vi "Measurement Logic.vi"() -> ()   [LabVIEW 2021, in "Efficiency And Load Regulation_PMIC.lvlib"]
uses:
  Efficiency And Load Regulation_PMIC.lvlib
  Measurement Configuration.ctl
  Measurement Results.ctl
  <vilib>/Plug-In SDKs/Measurements/Measure Call Context/Measure Call Context.lvclass
  <instrlib>/niDCPower/nidcpower.llb/niDCPower Sense.ctl
  <instrlib>/niDCPower/nidcpower.llb/niDCPower Source Mode.ctl
  <instrlib>/niDCPower/nidcpower.llb/niDCPower Wait For Event - Event.ctl
  <instrlib>/niDCPower/nidcpower.llb/niDCPower Output Function.ctl
  <instrlib>/niDCPower/nidcpower.llb/niDCPower Sequence Attribute Type.ctl
  <instrlib>/niDCPower/nidcpower.llb/niDCPower Get Channel Name From String.vi
  <instrlib>/niDCPower/nidcpower.llb/niDCPower Create Advanced Sequence Step With Channels.vi
  <instrlib>/niDCPower/nidcpower.llb/niDCPower Configure Digital Edge Source Trigger With Channels.vi
  <instrlib>/niDCPower/nidcpower.llb/niDCPower Configure Digital Edge Measure Trigger With Channels.vi
panel:
  out "measure call context out":refnum<class "Measure Call Context.lvclass">
  in  "measure call context in":refnum<class "Measure Call Context.lvclass">
  out "measurement results":T1
  in  "measurement configuration":T2={"Mode of operation"=enum."Perform measurement", "DUT setup time"=1.0, "Source delay"=0.005, "Aperture time"=0.005, "Nominal output voltage"=3.3, "Source resource name"="", "Source current limit"=25.0, "Source maximum power"=300.0, "Source start voltage"=5.0, "Source stop voltage"=20.0, "Source voltage sweep points"=10, "Load resource name"="", "Load voltage limit range"=6.0, "Load sweep type"="Logarithmic", "Load start current"=0.1, "Load stop current"=24.0, "Load current sweep points/points per decade"=10}
  out "error out":errorcluster
  in  "error in":errorcluster
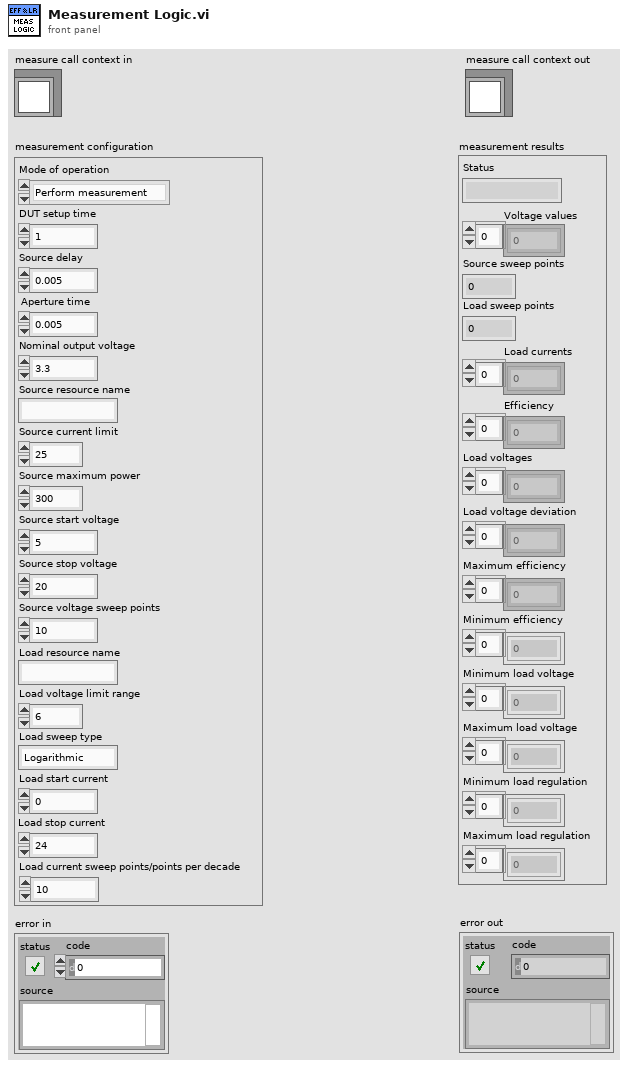
[diagram p1: front panel]
types:
  T1 = typedef "Efficiency And Load Regulation_PMIC.lvlib/Measurement Results.ctl" = cluster{"Status":string, "Voltage values":dbl[], "Source sweep points":i32, "Load sweep points":i32, "Load currents":dbl[], "Efficiency":dbl[], "Load voltages":dbl[], "Load voltage deviation":dbl[], "Maximum efficiency":dbl[], "Minimum efficiency":dbl[], "Minimum load voltage":dbl[], "Maximum load voltage":dbl[], "Minimum load regulation":dbl[], "Maximum load regulation":dbl[]}
  T2 = typedef "Efficiency And Load Regulation_PMIC.lvlib/Measurement Configuration.ctl" = cluster{"Mode of operation":enum32{"Power on the DUT", "Perform measurement", "Power off the DUT"}, "DUT setup time":dbl, "Source delay":dbl, "Aperture time":dbl, "Nominal output voltage":dbl, "Source resource name":string, "Source current limit":dbl, "Source maximum power":dbl, "Source start voltage":dbl, "Source stop voltage":dbl, "Source voltage sweep points":i32, "Load resource name":string, "Load voltage limit range":dbl, "Load sweep type":string, "Load start current":dbl, "Load stop current":dbl, "Load current sweep points/points per decade":i32}
  T3 = cluster{"Voltage values":dbl[], "Source out":refnum<k15>, "Source channel name":string, "Load out":refnum<k15>, "Load channel name":string, "Current values":dbl[], "Load sweep points":i32, "Source terminal name":string, "Measure terminal name":string, "Measurement Results":T1, "Source sequence name":string}
  T4 = enum32{"Power on the DUT", "Perform measurement", "Power off the DUT"}
  T5 = typedef "niDCPower Wait For Event - Event.ctl" = i32
  T6 = typedef "niDCPower Source Mode.ctl" = i32
  T7 = typedef "niDCPower Sense.ctl" = i32
  T8 = typedef "niDCPower Sequence Attribute Type.ctl" = i32
  T9 = typedef "niDCPower Output Function.ctl" = i32
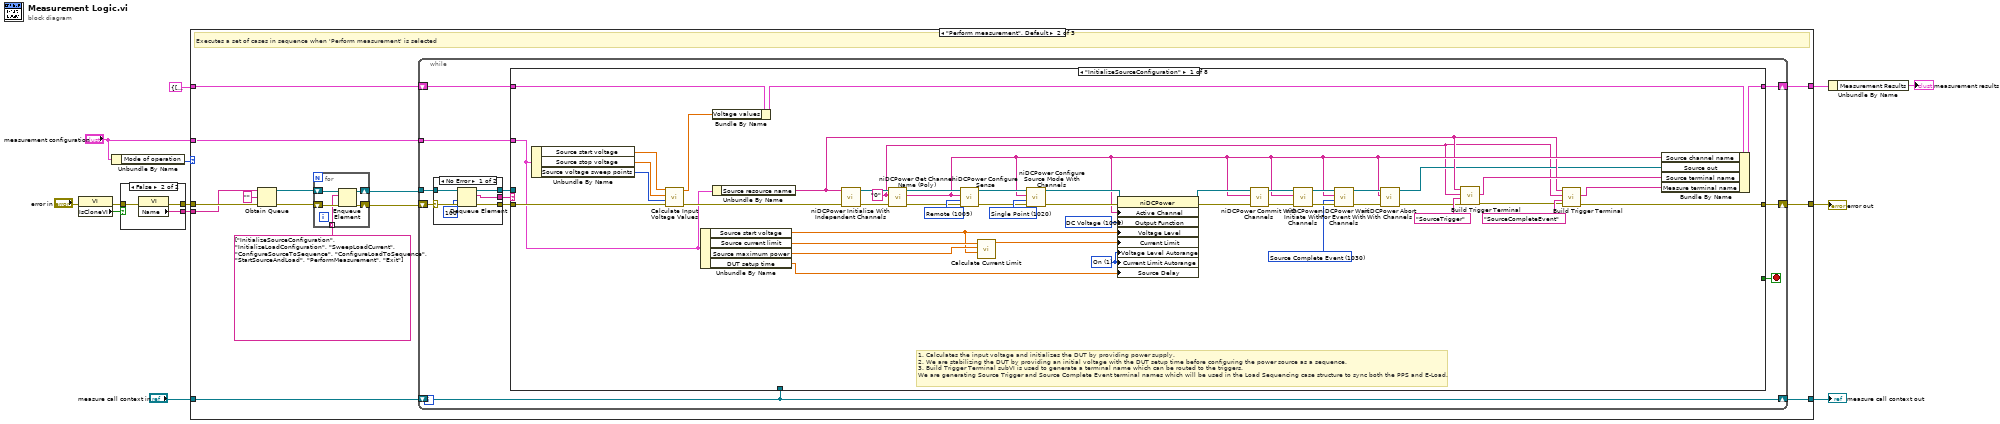
[diagram p0: block diagram]
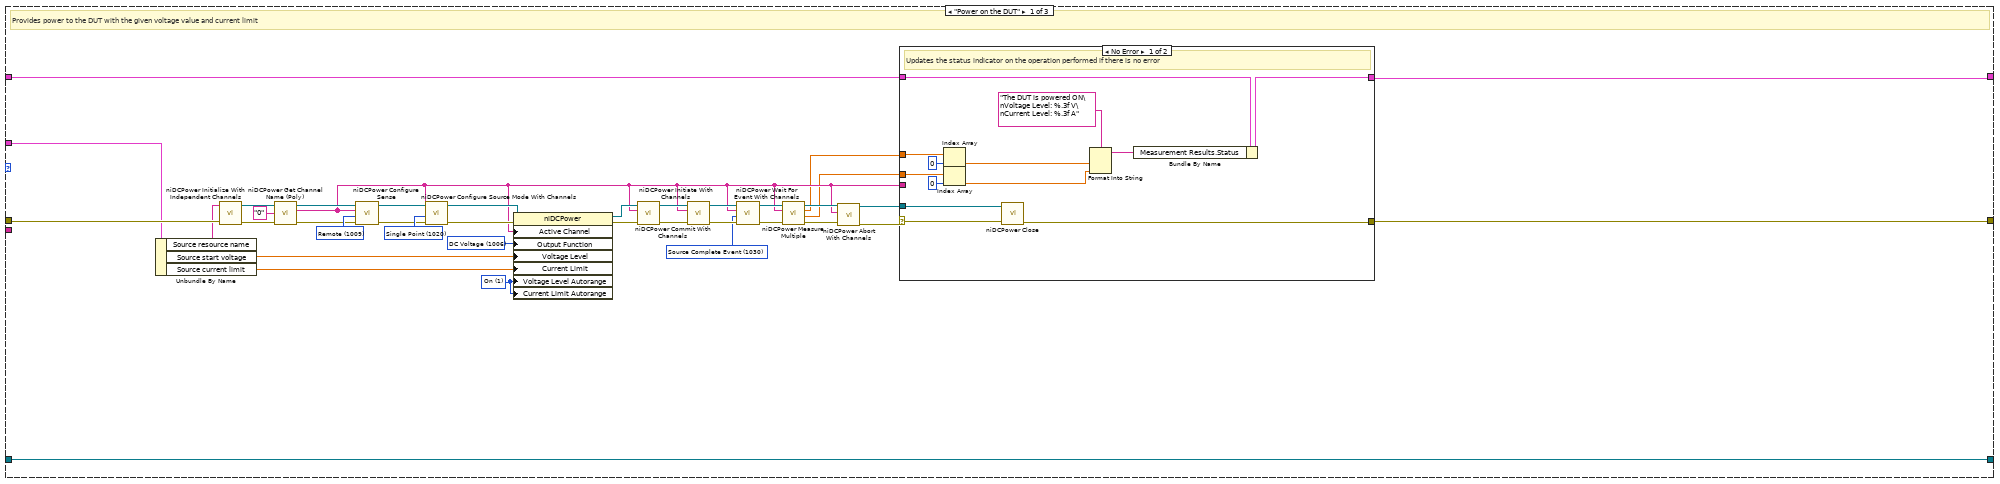
[diagram p2: hidden frame]
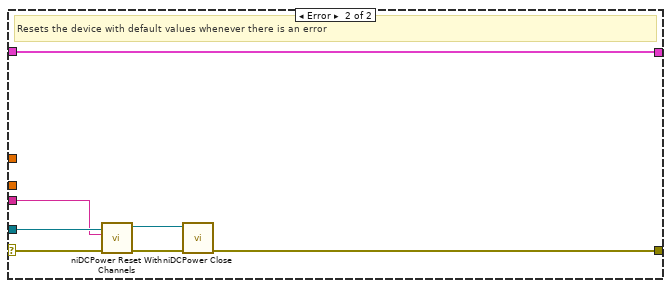
[diagram p3: hidden frame]
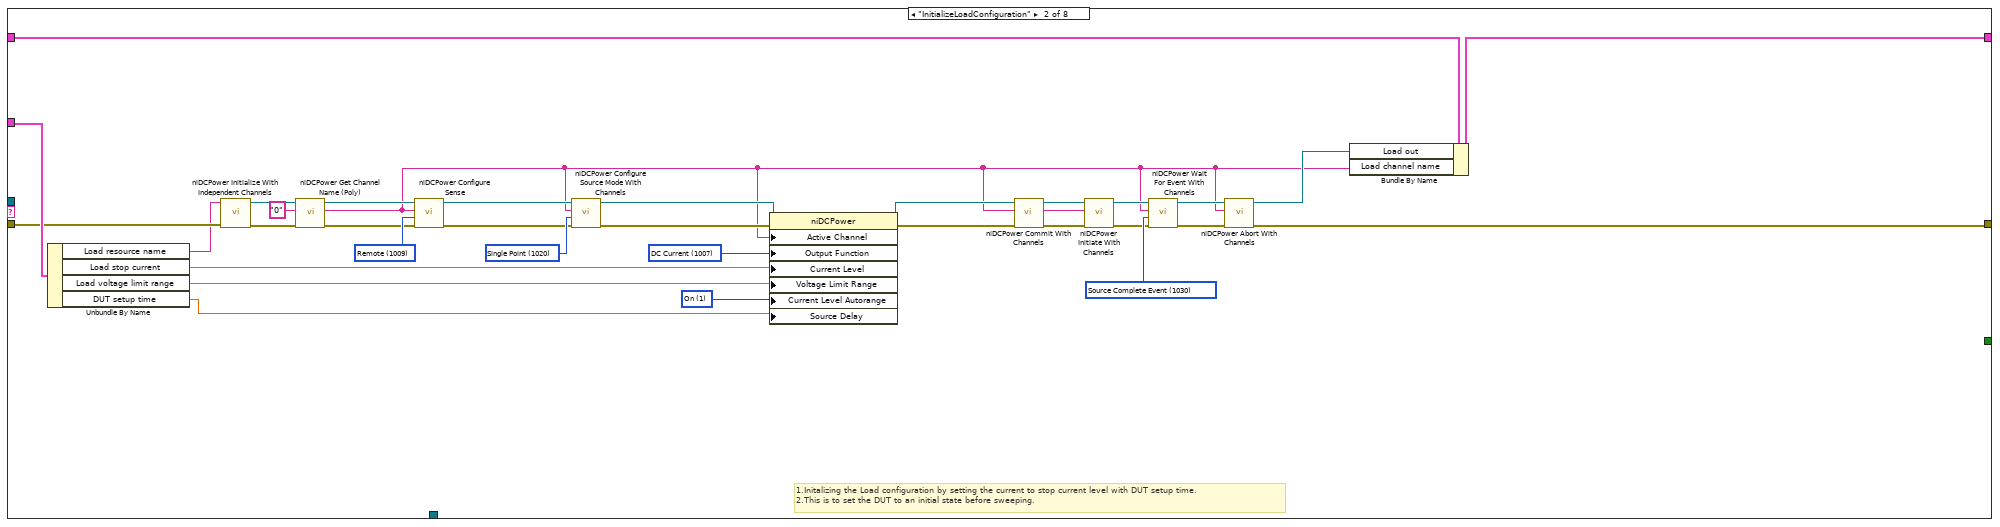
[diagram p4: hidden frame]
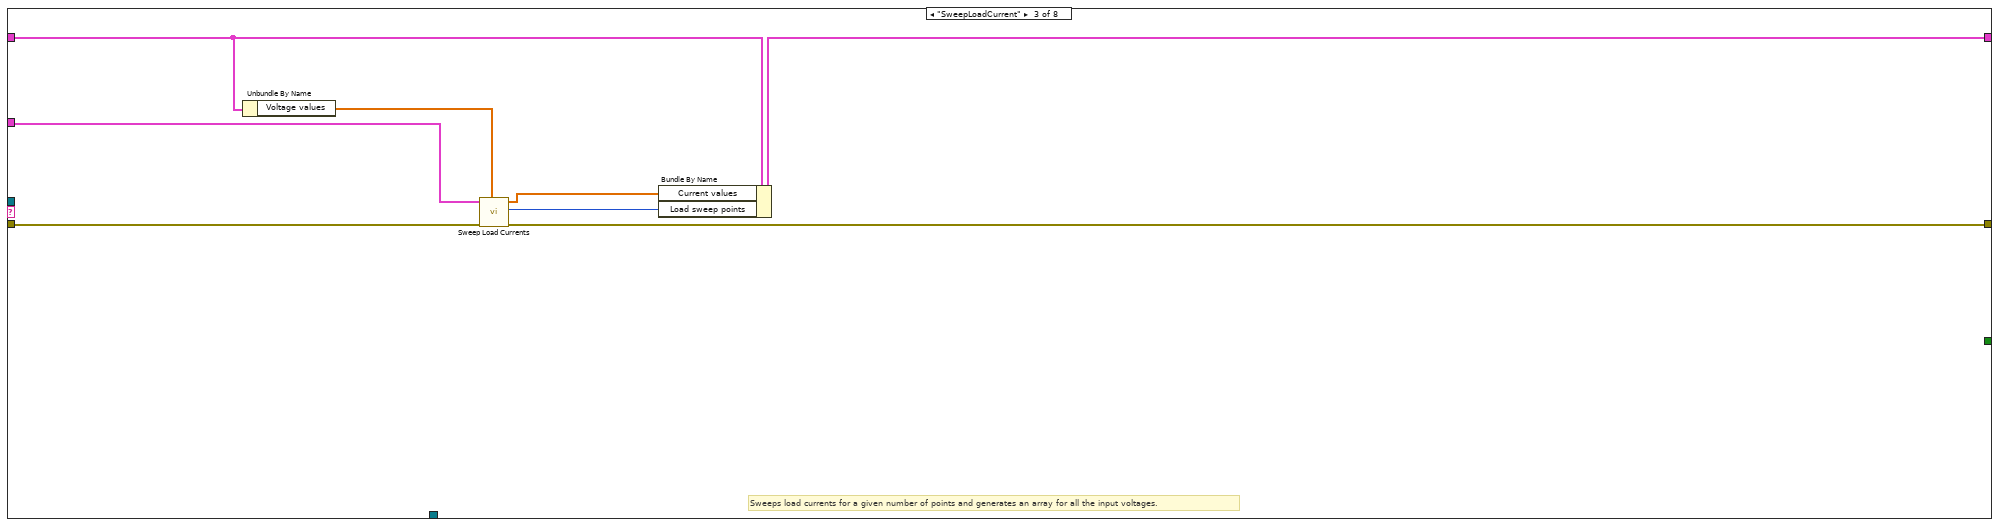
[diagram p5: hidden frame]
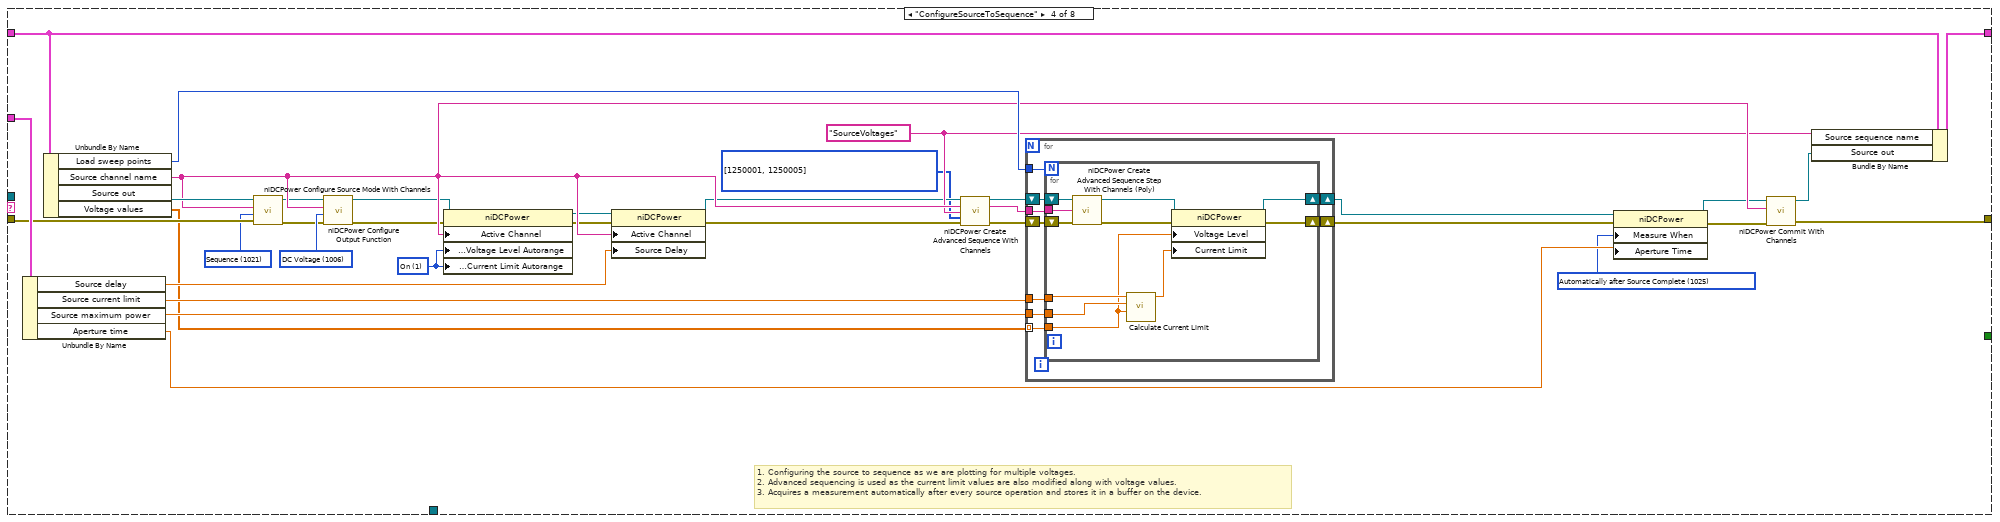
[diagram p6: hidden frame]
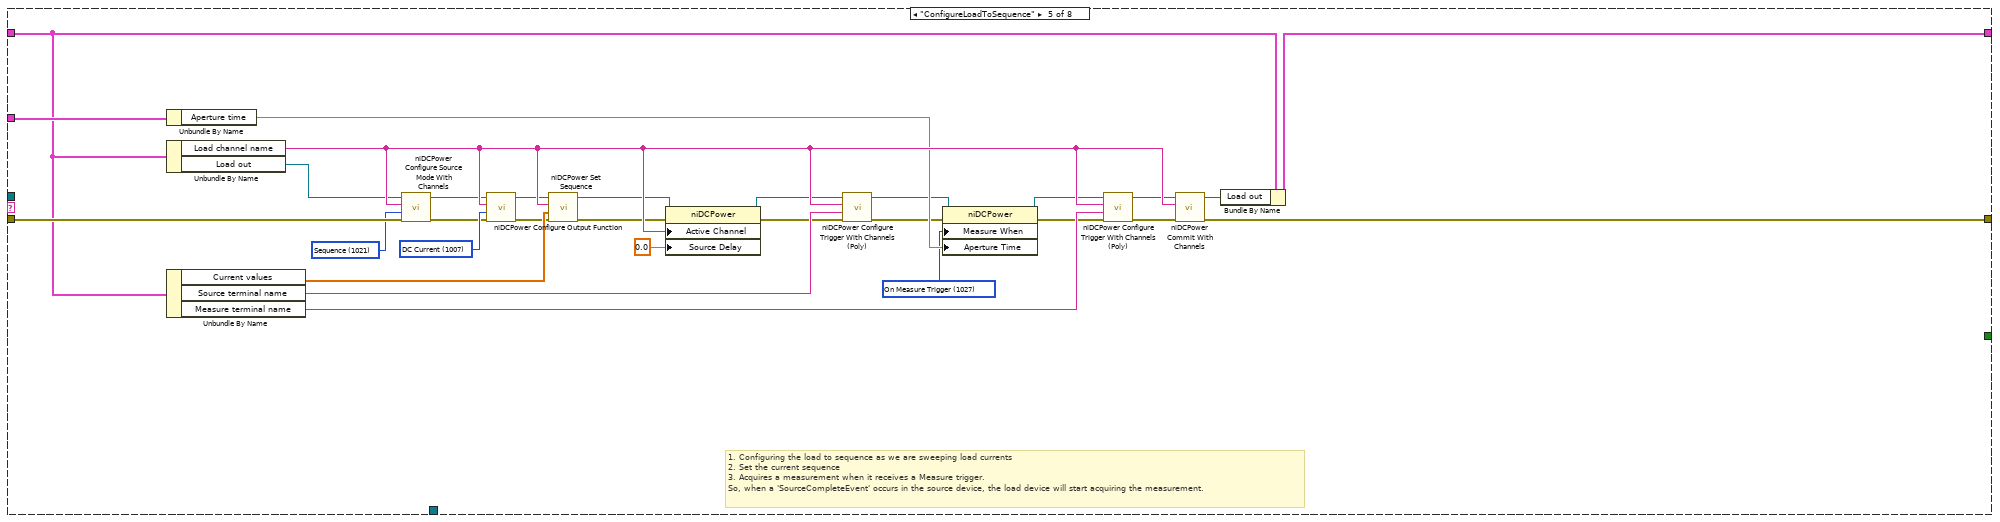
[diagram p7: hidden frame]
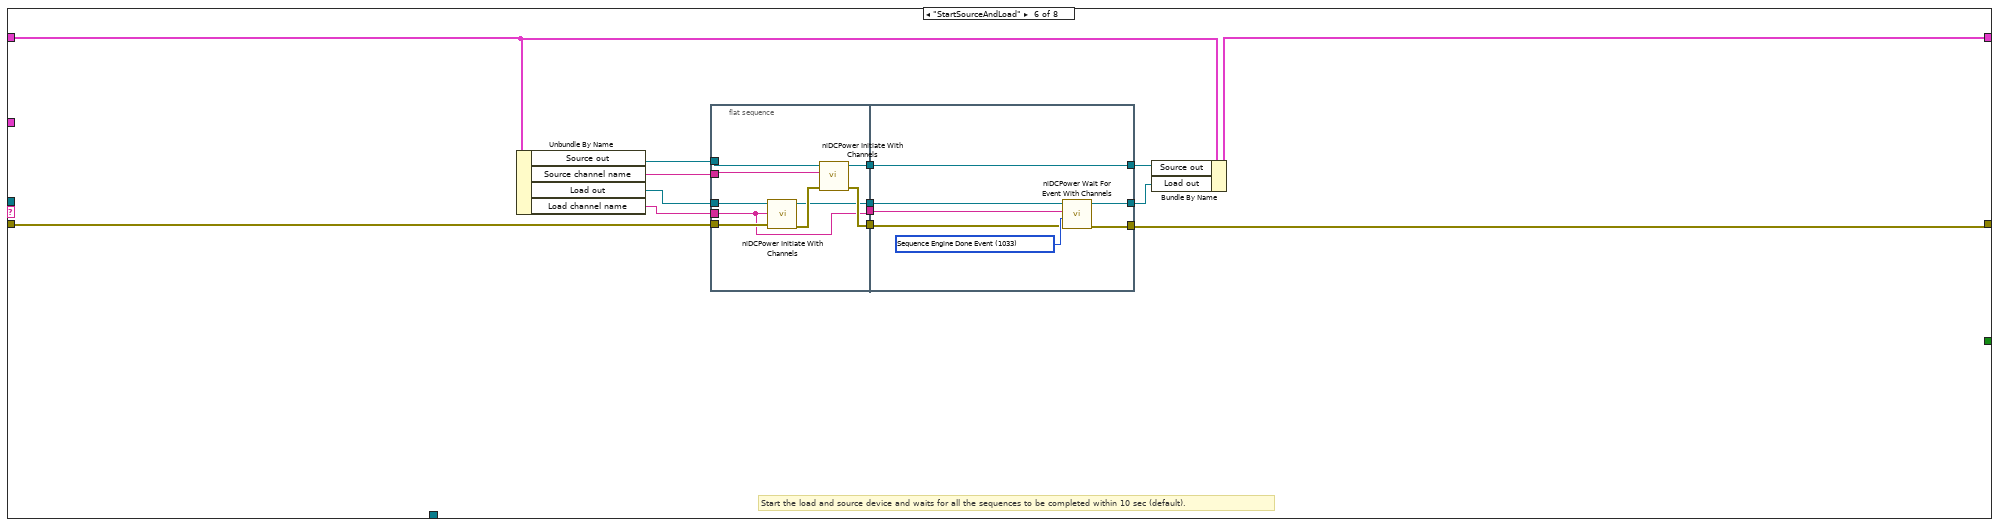
[diagram p8: hidden frame]
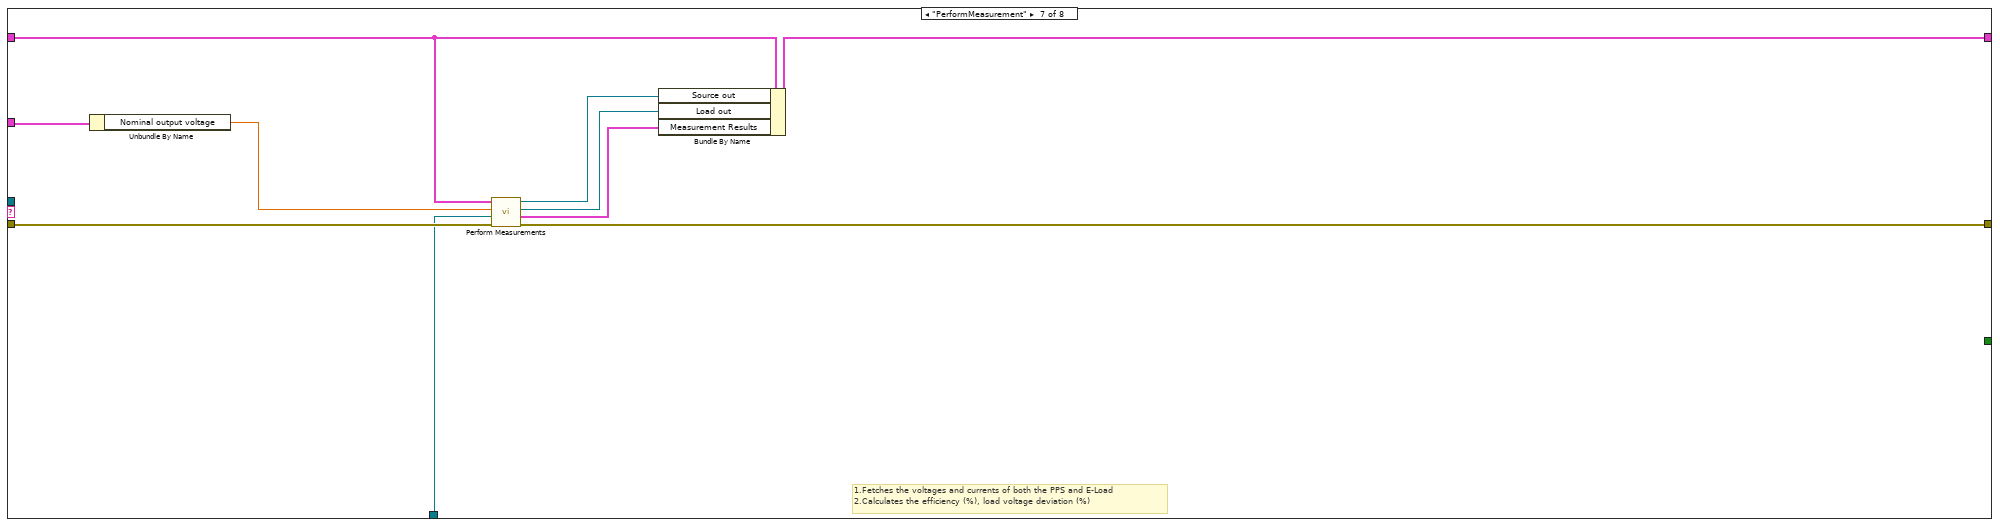
[diagram p9: hidden frame]
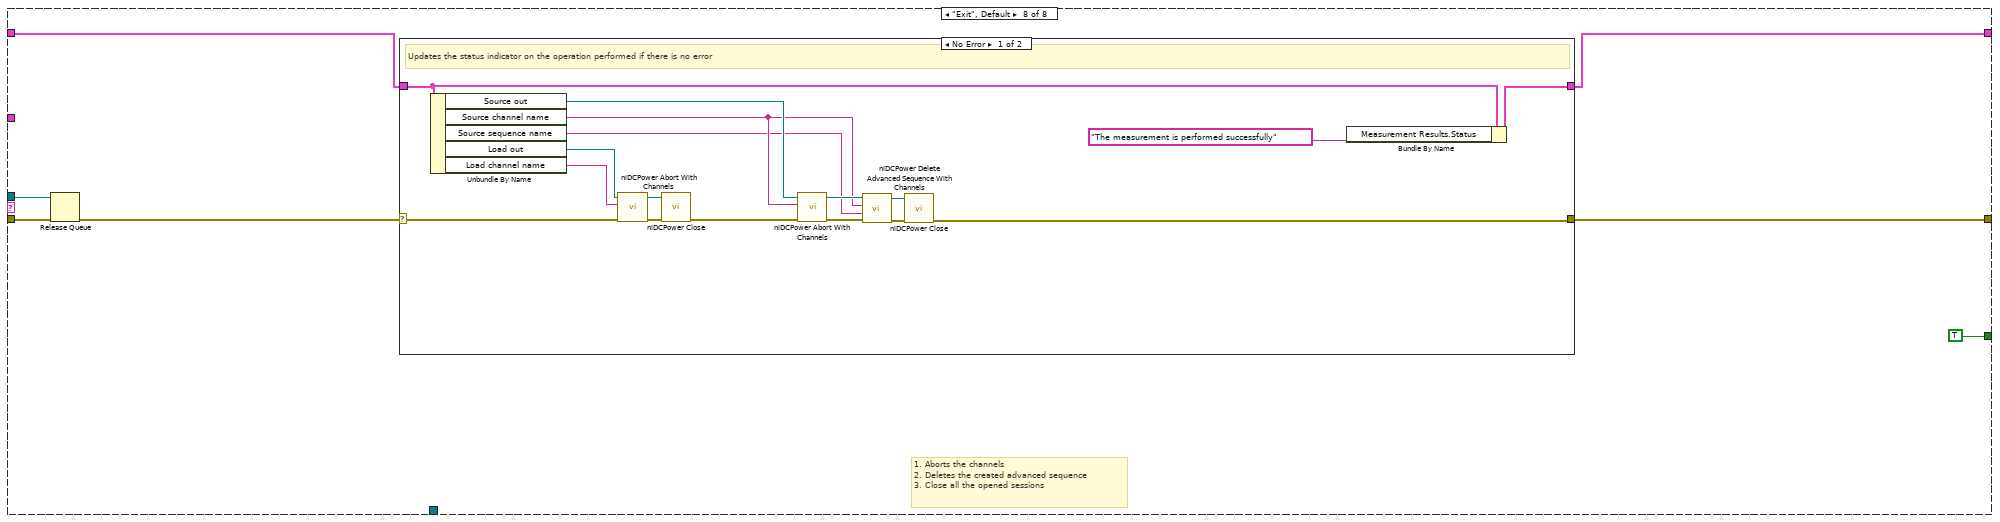
[diagram p10: hidden frame]
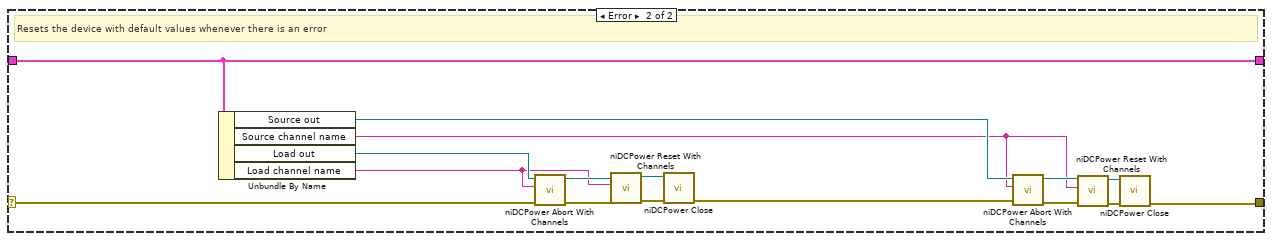
[diagram p11: hidden frame]
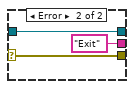
[diagram p12: hidden frame]
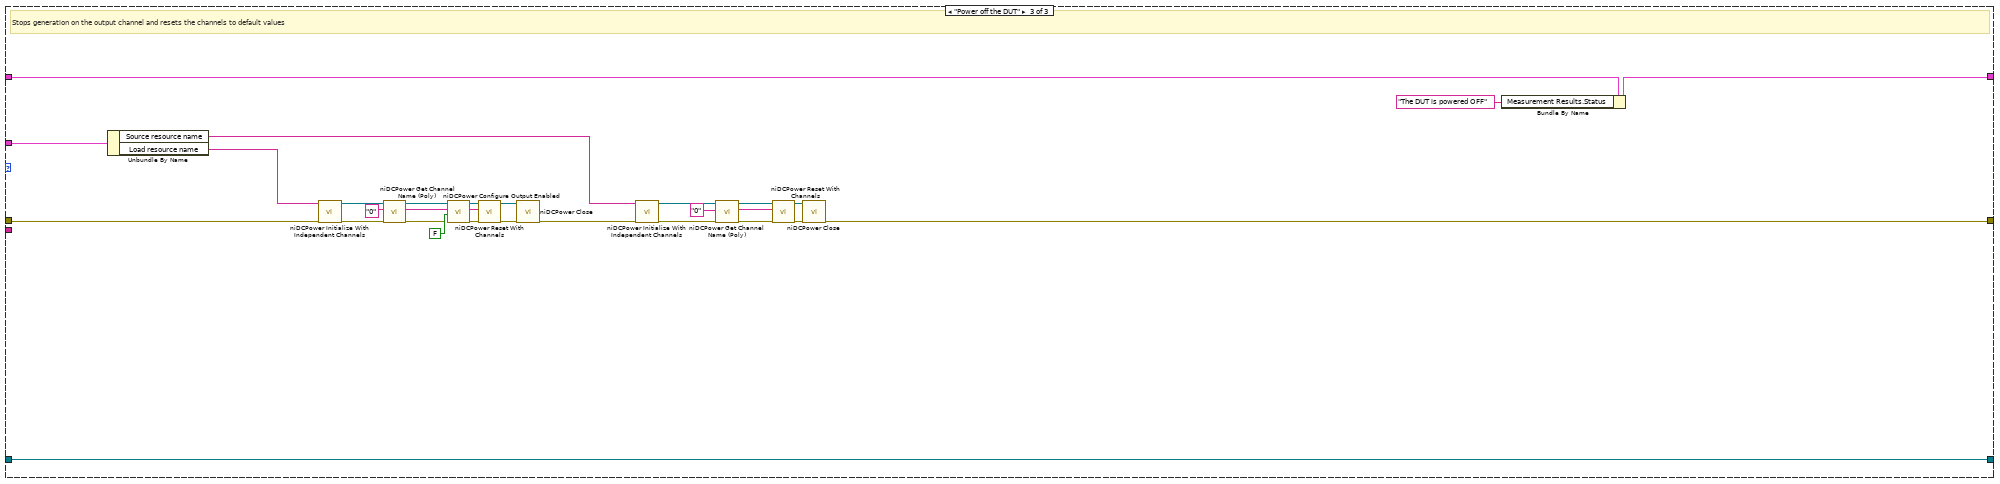
[diagram p13: hidden frame]
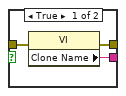
[diagram p14: hidden frame]
diagram:
  n1 = property class="VI"(error in="error in") -> (error out=w12:errorcluster, "IsCloneVI"=w13:bool)  [unwired: 1 in, 1 out]
  n2 = Unbundle By Name("measurement configuration") -> ("Mode of operation"=w5:T4)
  n3 = case shown="False" w13 {
    tunnel: [w16 w19] -> w7
    tunnel: [w15 w18] -> w6
    tunnel: w12 -> [w14 w17]
    frame True {
      n4 = property class="VI"(error in=w14) -> (error out=w16:errorcluster, "Clone Name"=w15:string)  [unwired: 1 in, 1 out]
    }
    frame False {
      n5 = property class="VI"(error in=w17) -> (error out=w19:errorcluster, "Name"=w18:string)  [unwired: 1 in, 1 out]
    }
  }
  n6 = case shown="\"Perform measurement\", Default" w5 {
    tunnel: [w21 w77 w385] -> w1
    tunnel: w7 -> [w37 w87 w384]
    tunnel: w6 -> [_ w86 _]
    tunnel: "measurement configuration" -> [w30 w83 w372]
    tunnel: [w22 w78 w368] -> w2
    tunnel: T3 {"Voltage values"=[], "Source out"="", "Source channel name"="", "Load out"="", "Load channel name"="", "Current values"=[], "Load sweep points"=0, "Source terminal name"="", "Measure terminal name"="", "Measurement Results"={"Status"="", "Voltage values"=[], "Source sweep points"=0, "Load sweep points"=0, "Load currents"=[], "Efficiency"=[], "Load voltages"=[], "Load voltage deviation"=[], "Maximum efficiency"=[], "Minimum efficiency"=[], "Minimum load voltage"=[], "Maximum load voltage"=[], "Minimum load regulation"=[], "Maximum load regulation"=[]}, "Source sequence name"=""} -> [w23 w82 w370]
    tunnel: "measure call context in" -> [w20 w80 w371]
    tunnel: [w20 w79 w371] -> w3
    frame "Power on the DUT" {
      w40 = 1 items=["Off", "On"] ("Source:DC Voltage:Voltage Level Autorange")
      w41 = T5 1030 items=["Source Complete Event"=1030, "Measure Complete Event"=1031, "Sequence Iteration Complete Event"=1032, "Sequence Engine Done Event"=1033, "Pulse Complete Event"=1051, "Ready For Pulse Trigger Event"=1052] ("event")
      w52 = T6 1020 items=["Single Point"=1020, "Sequence"=1021] ("source mode")
      w47 = 1006 items=["DC Voltage"=1006, "DC Current"=1007, "Pulse Voltage"=1049, "Pulse Current"=1050] ("Source:Output Function")
      w42 = T7 1009 items=["Local"=1008, "Remote"=1009] ("sense")
      # "Provides power to the DUT with the given voltage value and current limit"
      n7 = Unbundle By Name(w30) -> ("Source resource name"=w34:string, "Source start voltage"=w29:dbl, "Source current limit"=w35:dbl)
      n8 = call <instrlib>:"niDCPower Initialize With Independent Channels.vi"("error in (no error)"=w37, "resource name"=w34) -> ("error out"=w39:errorcluster, "instrument handle out"=w43:refnum<k15>)  [unwired: 8 in]
      n9 = call-poly <instrlib>:"niDCPower Get Channel Name (Poly).vi"("index"="0", "instrument handle"=w43) -> ("name"=w26:string, "instrument handle out"=w38:refnum<k15>)  [unwired: 7 in, 1 out]
      n10 = call <instrlib>:"niDCPower Configure Sense.vi"("error in (no error)"=w39, "sense"=w42, "channel name"=w26, "instrument handle"=w38) -> ("error out"=w50:errorcluster, "instrument handle out"=w48:refnum<k15>)  [unwired: 6 in]
      n11 = call <instrlib>:"niDCPower Configure Source Mode With Channels.vi"("error in (no error)"=w50, "source mode"=w52, "channel name"=w26, "instrument handle"=w48) -> ("error out"=w51:errorcluster, "instrument handle out"=w49:refnum<k15>)  [unwired: 6 in]
      n12 = property class="niDCPower"(reference=w49, error in=w51, "Active Channel"=w26, "Output Function"=w47, "Voltage Level"=w29, "Current Limit"=w35, "Voltage Level Autorange"=w40, "Current Limit Autorange"=w40) -> (reference out=w53:refnum<k15>, error out=w54:errorcluster)
      n13 = call <instrlib>:"niDCPower Commit With Channels.vi"("error in (no error)"=w54, "channel name"=w26, "instrument handle"=w53) -> ("error out"=w56:errorcluster, "instrument handle out"=w55:refnum<k15>)  [unwired: 7 in]
      n14 = call <instrlib>:"niDCPower Initiate With Channels.vi"("error in (no error)"=w56, "channel name"=w26, "instrument handle"=w55) -> ("error out"=w44:errorcluster, "instrument handle out"=w45:refnum<k15>)  [unwired: 7 in]
      n15 = call <instrlib>:"niDCPower Wait For Event With Channels.vi"("error in (no error)"=w44, "event"=w41, "channel name"=w26, "instrument handle"=w45) -> ("error out"=w32:errorcluster, "instrument handle out"=w46:refnum<k15>)  [unwired: 6 in]
      n16 = call <instrlib>:"niDCPower Measure Multiple.vi"("error in (no error)"=w32, "channel name"=w26, "instrument handle"=w46) -> ("error out"=w31:errorcluster, "current measurements"=w24:dbl[], "voltage measurements"=w25:dbl[], "instrument handle out"=w33:refnum<k15>)  [unwired: 5 in]
      n17 = call <instrlib>:"niDCPower Abort With Channels.vi"("error in (no error)"=w31, "channel name"=w26, "instrument handle"=w33) -> ("error out"=w28:errorcluster, "instrument handle out"=w27:refnum<k15>)  [unwired: 7 in]
      n18 = case shown="No Error" w28 {
        selector: w28 -> [w69 w74]
        tunnel: [w68 w73] -> w21
        tunnel: [w67 w70] -> w22
        tunnel: w27 -> [w62 w72]
        tunnel: w26 -> [_ w71]
        tunnel: w25 -> [w61 _]
        tunnel: w24 -> [w60 _]
        tunnel: w23 -> [w59 w70]
        frame No Error {
          # "Updates the status indicator on the operation performed if there is no error"
          n19 = Index Array(array=w61, index=0) -> (element=w58:dbl)
          n20 = Index Array(array=w60, index=0) -> (element=w57:dbl)
          n21 = call <instrlib>:"niDCPower Close.vi"("error in (no error)"=w69, "instrument handle"=w62) -> ("error out"=w68:errorcluster)  [unwired: 9 out]
          n22 = Format Into String(format string="The DUT is powered ON\nVoltage Level: %.3f V\nCurrent Level: %.3f A" ("message"), w58, w57) -> (resulting string=w65:string)  [unwired: 2 in, 1 out]
          n23 = Bundle By Name(cluster=w59, "Measurement Results.Status"=w65) -> (w67:T3)
        }
        frame Error {
          # "Resets the device with default values whenever there is an error"
          n24 = call <instrlib>:"niDCPower Reset With Channels.vi"("error in (no error)"=w74, "channel name"=w71, "instrument handle"=w72) -> ("error out"=w76:errorcluster, "instrument handle out"=w75:refnum<k15>)  [unwired: 7 in]
          n25 = call <instrlib>:"niDCPower Close.vi"("error in (no error)"=w76, "instrument handle"=w75) -> ("error out"=w73:errorcluster)  [unwired: 9 out]
        }
      }
    }
    frame "Perform measurement", Default {
      # "Executes a set of cases in sequence when 'Perform measurement' is selected"
      n26 = Obtain Queue(name (unnamed)=w86, element data type="", error in (no error)=w87) -> (queue out=w89:refnum<queue>, error out=w90:errorcluster)  [unwired: 2 in, 1 out]
      n27 = for {
        shift-right: [w365] -> w84
        shift-left: w89 -> [w367]
        shift-right: [w364] -> w81
        shift-left: w90 -> [w366]
        tunnel: string[] ["InitializeSourceConfiguration", "InitializeLoadConfiguration", "SweepLoadCurrent", "ConfigureSourceToSequence", "ConfigureLoadToSequence", "StartSourceAndLoad", "PerformMeasurement", "Exit"] ("Step sequence") -> [w363] mode=indexing
        n28 = Enqueue Element(queue=w367, element=w363, error in (no error)=w366) -> (queue out=w365:refnum<queue>, error out=w364:errorcluster)  [unwired: 1 in, 1 out]
      }
      n29 = while {
        tunnel: w84 -> [w101]
        tunnel: w83 -> [w97]
        shift-right: [w94] -> w78
        shift-left: w82 -> [w95]
        shift-right: [w93] -> w77
        shift-left: w81 -> [w100]
        shift-right: [w92] -> w79
        shift-left: w80 -> [w92]
        stop <- w91 stop-if-true
        n30 = case shown="No Error" w100 {
          selector: w100 -> [w357 w361]
          tunnel: w101 -> [w359 w360]
          tunnel: [w358 "Exit" ("t")] -> w99
          tunnel: [w356 w361] -> w96
          tunnel: [w354 w360] -> w98
          frame No Error {
            n31 = Dequeue Element(queue=w359, timeout in ms (-1)=100, error in (no error)=w357) -> (queue out=w354:refnum<queue>, element=w358:string, error out=w356:errorcluster)  [unwired: 1 out]
          }
          frame Error {
          }
        }
        n32 = case shown="\"InitializeSourceConfiguration\"" w99 {
          tunnel: w98 -> [_ _ _ _ _ _ _ w315]
          tunnel: w97 -> [w118 w181 w182 w221 w267 _ w311 _]
          tunnel: w96 -> [w127 w180 w187 w220 w273 w279 w313 w320]
          tunnel: w95 -> [w147 w155 w188 w223 w263 w278 w306 w318]
          tunnel: [w148 w175 w189 w222 w262 w275 w304 w316] -> w94
          tunnel: [w108 w179 w186 w211 w265 w274 w312 w317] -> w93
          tunnel: w92 -> [_ _ _ _ _ _ w305 _]
          tunnel: [_ _ _ _ _ _ _ TRUE] -> w91
          frame "InitializeSourceConfiguration" {
            w103 = "0" ("index")
            w129 = 1 items=["Off", "On"] ("Source:DC Voltage:Voltage Level Autorange")
            w130 = T5 1030 items=["Source Complete Event"=1030, "Measure Complete Event"=1031, "Sequence Iteration Complete Event"=1032, "Sequence Engine Done Event"=1033, "Pulse Complete Event"=1051, "Ready For Pulse Trigger Event"=1052] ("event")
            w142 = T6 1020 items=["Single Point"=1020, "Sequence"=1021] ("source mode")
            w137 = 1006 items=["DC Voltage"=1006, "DC Current"=1007, "Pulse Voltage"=1049, "Pulse Current"=1050] ("Source:Output Function")
            w131 = T7 1009 items=["Local"=1008, "Remote"=1009] ("sense")
            # "1. Calculates the input voltage and initializes the DUT by providing power supply.\n2. We are stabilizing the DUT by providing an initial voltage with the DUT setup time before configuring the power source as a sequence.\n3. Build Trigger Terminal subVI is used to generate a terminal name which can be routed to the triggers. \nWe are generating Source Trigger and Source Complete Event terminal names which will be used in the Load Sequencing case structure to sync both the PPS and E-Load."
            n33 = Unbundle By Name(w118) -> ("Source start voltage"=w124:dbl, "Source stop voltage"=w123:dbl, "Source voltage sweep points"=w122:i32)
            n34 = call "Calculate Input Voltage Values.vi"("error in"=w127, "Points"=w122, "Voltage stop level"=w123, "Voltage start level"=w124) -> ("error out"=w126:errorcluster, "Voltage values"=w125:dbl[])  [unwired: 6 in]
            n35 = Unbundle By Name(w118) -> ("Source start voltage"=w102:dbl, "Source current limit"=w121:dbl, "Source maximum power"=w120:dbl, "DUT setup time"=w128:dbl)
            n36 = Bundle By Name(cluster=w147, "Voltage values"=w125) -> (w117:T3)
            n37 = Unbundle By Name(w118) -> ("Source resource name"=w105:string)
            n38 = call <instrlib>:"niDCPower Initialize With Independent Channels.vi"("error in (no error)"=w126, "resource name"=w105) -> ("error out"=w114:errorcluster, "instrument handle out"=w132:refnum<k15>)  [unwired: 8 in]
            n39 = call-poly <instrlib>:"niDCPower Get Channel Name (Poly).vi"("error in (no error)"=w114, "index"=w103, "instrument handle"=w132) -> ("error out"=w113:errorcluster, "name"=w115:string, "instrument handle out"=w116:refnum<k15>)  [unwired: 6 in]
            n40 = call <instrlib>:"niDCPower Configure Sense.vi"("error in (no error)"=w113, "sense"=w131, "channel name"=w115, "instrument handle"=w116) -> ("error out"=w140:errorcluster, "instrument handle out"=w138:refnum<k15>)  [unwired: 6 in]
            n41 = call "Calculate Current Limit.vi"("Voltage value"=w102, "Maximum power"=w120, "Current limit in"=w121) -> ("Current limit out"=w119:dbl)  [unwired: 8 in]
            n42 = call <instrlib>:"niDCPower Configure Source Mode With Channels.vi"("error in (no error)"=w140, "source mode"=w142, "channel name"=w115, "instrument handle"=w138) -> ("error out"=w141:errorcluster, "instrument handle out"=w139:refnum<k15>)  [unwired: 6 in]
            n43 = property class="niDCPower"(reference=w139, error in=w141, "Active Channel"=w115, "Output Function"=w137, "Voltage Level"=w102, "Current Limit"=w119, "Voltage Level Autorange"=w129, "Current Limit Autorange"=w129, "Source Delay"=w128) -> (reference out=w143:refnum<k15>, error out=w144:errorcluster)
            n44 = call <instrlib>:"niDCPower Commit With Channels.vi"("error in (no error)"=w144, "channel name"=w115, "instrument handle"=w143) -> ("error out"=w146:errorcluster, "instrument handle out"=w145:refnum<k15>)  [unwired: 7 in]
            n45 = call <instrlib>:"niDCPower Initiate With Channels.vi"("error in (no error)"=w146, "channel name"=w115, "instrument handle"=w145) -> ("error out"=w133:errorcluster, "instrument handle out"=w134:refnum<k15>)  [unwired: 7 in]
            n46 = call <instrlib>:"niDCPower Wait For Event With Channels.vi"("error in (no error)"=w133, "event"=w130, "channel name"=w115, "instrument handle"=w134) -> ("error out"=w136:errorcluster, "instrument handle out"=w135:refnum<k15>)  [unwired: 6 in]
            n47 = call <instrlib>:"niDCPower Abort With Channels.vi"("error in (no error)"=w136, "channel name"=w115, "instrument handle"=w135) -> ("error out"=w110:errorcluster, "instrument handle out"=w104:refnum<k15>)  [unwired: 7 in]
            n48 = call "Build Trigger Terminal.vi"("error in (no error)"=w110, "Trigger/Event Name"="SourceTrigger", "Channel Name"=w103, "Resource Name"=w105) -> ("error out"=w109:errorcluster, "Terminal Name"=w107:string)  [unwired: 6 in]
            n49 = call "Build Trigger Terminal.vi"("error in (no error)"=w109, "Trigger/Event Name"="SourceCompleteEvent", "Channel Name"=w103, "Resource Name"=w105) -> ("error out"=w108:errorcluster, "Terminal Name"=w106:string)  [unwired: 6 in]
            n50 = Bundle By Name(cluster=w117, "Source channel name"=w115, "Source out"=w104, "Source terminal name"=w107, "Measure terminal name"=w106) -> (w148:T3)
          }
          frame "InitializeLoadConfiguration" {
            w170 = T6 1020 items=["Single Point"=1020, "Sequence"=1021] ("source mode")
            w163 = T5 1030 items=["Source Complete Event"=1030, "Measure Complete Event"=1031, "Sequence Iteration Complete Event"=1032, "Sequence Engine Done Event"=1033, "Pulse Complete Event"=1051, "Ready For Pulse Trigger Event"=1052] ("event")
            w157 = 1 items=["Off", "On"] ("Source:DC Current:Current Level Autorange")
            w159 = 1007 items=["DC Voltage"=1006, "DC Current"=1007, "Pulse Voltage"=1049, "Pulse Current"=1050] ("Source:Output Function")
            w158 = T7 1009 items=["Local"=1008, "Remote"=1009] ("sense")
            # "1.Initalizing the Load configuration by setting the current to stop current level with DUT setup time.\n2.This is to set the DUT to an initial state before sweeping."
            n51 = Unbundle By Name(w181) -> ("Load resource name"=w177:string, "Load stop current"=w149:dbl, "Load voltage limit range"=w178:dbl, "DUT setup time"=w156:dbl)
            n52 = call <instrlib>:"niDCPower Initialize With Independent Channels.vi"("error in (no error)"=w180, "resource name"=w177) -> ("error out"=w151:errorcluster, "instrument handle out"=w160:refnum<k15>)  [unwired: 8 in]
            n53 = call-poly <instrlib>:"niDCPower Get Channel Name (Poly).vi"("error in (no error)"=w151, "index"="0", "instrument handle"=w160) -> ("error out"=w150:errorcluster, "name"=w152:string, "instrument handle out"=w154:refnum<k15>)  [unwired: 6 in]
            n54 = call <instrlib>:"niDCPower Configure Sense.vi"("error in (no error)"=w150, "sense"=w158, "channel name"=w152, "instrument handle"=w154) -> ("error out"=w167:errorcluster, "instrument handle out"=w166:refnum<k15>)  [unwired: 6 in]
            n55 = call <instrlib>:"niDCPower Configure Source Mode With Channels.vi"("error in (no error)"=w167, "source mode"=w170, "channel name"=w152, "instrument handle"=w166) -> ("error out"=w169:errorcluster, "instrument handle out"=w168:refnum<k15>)  [unwired: 6 in]
            n56 = property class="niDCPower"(reference=w168, error in=w169, "Active Channel"=w152, "Output Function"=w159, "Current Level"=w149, "Voltage Limit Range"=w178, "Current Level Autorange"=w157, "Source Delay"=w156) -> (reference out=w171:refnum<k15>, error out=w172:errorcluster)
            n57 = call <instrlib>:"niDCPower Commit With Channels.vi"("error in (no error)"=w172, "channel name"=w152, "instrument handle"=w171) -> ("error out"=w173:errorcluster, "instrument handle out"=w174:refnum<k15>)  [unwired: 7 in]
            n58 = call <instrlib>:"niDCPower Initiate With Channels.vi"("error in (no error)"=w173, "channel name"=w152, "instrument handle"=w174) -> ("error out"=w161:errorcluster, "instrument handle out"=w162:refnum<k15>)  [unwired: 7 in]
            n59 = call <instrlib>:"niDCPower Wait For Event With Channels.vi"("error in (no error)"=w161, "event"=w163, "channel name"=w152, "instrument handle"=w162) -> ("error out"=w165:errorcluster, "instrument handle out"=w164:refnum<k15>)  [unwired: 6 in]
            n60 = call <instrlib>:"niDCPower Abort With Channels.vi"("error in (no error)"=w165, "channel name"=w152, "instrument handle"=w164) -> ("error out"=w179:errorcluster, "instrument handle out"=w176:refnum<k15>)  [unwired: 7 in]
            n61 = Bundle By Name(cluster=w155, "Load out"=w176, "Load channel name"=w152) -> (w175:T3)
          }
          frame "SweepLoadCurrent" {
            # "Sweeps load currents for a given number of points and generates an array for all the input voltages."
            n62 = Unbundle By Name(w188) -> ("Voltage values"=w183:dbl[])
            n63 = call "Sweep Load Currents.vi"("Voltage values"=w183, "error in"=w187, "Measurement Configuration"=w182) -> ("error out"=w186:errorcluster, "Load sweep points"=w185:i32, "Current values"=w184:dbl[])  [unwired: 6 in]
            n64 = Bundle By Name(cluster=w188, "Current values"=w184, "Load sweep points"=w185) -> (w189:T3)
          }
          frame "ConfigureSourceToSequence" {
            w193 = 1025 items=["Automatically after Source Complete"=1025, "On Demand"=1026, "On Measure Trigger"=1027] ("Measurement:Advanced:Measure When")
            w201 = 1 items=["Off", "On"] ("DC Voltage:Voltage Level Autorange")
            w200 = T8[] [1250001, 1250005] items=["Source -> Output Function"=1150008, "Source -> Output Enabled"=1250006, "Source -> Output Resistance"=1150061, "Source -> Transient Response"=1150062, "Source -> Custom Transient Response -> Voltage Gain Bandwidth"=1150067, "Source -> Custom Transient Response -> Voltage Compensation Frequency"=1150068, "Source -> Custom Transient Response -> Voltage Pole-Zero Ratio"=1150069, "Source -> Custom Transient Response -> Current Gain Bandwidth"=1150070, "Source -> Custom Transient Response -> Current Compensation Frequency"=1150071, "Source -> Custom Transient Response -> Current Pole-Zero Ratio"=1150072, "Source -> DC Voltage -> Voltage Level"=1250001, "Source -> DC Voltage -> Voltage Level Range"=1150005, "Source -> DC Voltage -> Current Limit"=1250005, "Source -> DC Voltage -> Current Limit High"=1150187, "Source -> DC Voltage -> Current Limit Low"=1150188, "Source -> DC Voltage -> Current Limit Range"=1150004, "Source -> DC Current -> Current Level"=1150009, "Source -> DC Current -> Current Level Range"=1150011, "Source -> DC Current -> Voltage Limit"=1150010, "Source -> DC Current -> Voltage Limit High"=1150185, "Source -> DC Current -> Voltage Limit Low"=1150186, "Source -> DC Current -> Voltage Limit Range"=1150012, "Source -> Pulse Voltage -> Pulse Voltage Level"=1150080, "Source -> Pulse Voltage -> Pulse Bias Voltage Level"=1150082, "Source -> Pulse Voltage -> Pulse Voltage Level Range"=1150084, "Source -> Pulse Voltage -> Pulse Current Limit"=1150081, "Source -> Pulse Voltage -> Pulse Current Limit High"=1150193, "Source -> Pulse Voltage -> Pulse Current Limit Low"=1150194, "Source -> Pulse Voltage -> Pulse Bias Current Limit"=1150083, "Source -> Pulse Voltage -> Pulse Bias Current Limit High"=1150195, "Source -> Pulse Voltage -> Pulse Bias Current Limit Low"=1150196, "Source -> Pulse Voltage -> Pulse Current Limit Range"=1150085, "Source -> Pulse Current -> Pulse Current Level"=1150086, "Source -> Pulse Current -> Pulse Bias Current Level"=1150088, "Source -> Pulse Current -> Pulse Current Level Range"=1150090, "Source -> Pulse Current -> Pulse Voltage Limit"=1150087, "Source -> Pulse Current -> Pulse Voltage Limit High"=1150189, "Source -> Pulse Current -> Pulse Voltage Limit Low"=1150190, "Source -> Pulse Current -> Pulse Bias Voltage Limit"=1150089, "Source -> Pulse Current -> Pulse Bias Voltage Limit High"=1150191, "Source -> Pulse Current -> Pulse Bias Voltage Limit Low"=1150192, "Source -> Pulse Current -> Pulse Voltage Limit Range"=1150091, "Source -> Advanced -> Source Delay"=1150051, "Source -> Advanced -> Pulse Bias Delay"=1150092, "Source -> Advanced -> Pulse On Time"=1150093, "Source -> Advanced -> Pulse Off Time"=1150094, "Source -> Advanced -> OVP Enabled"=1250002, "Source -> Advanced -> OVP Limit"=1250003, "Source -> Advanced -> Compliance Limit Symmetry"=1150184, "Source -> Advanced -> Sequence Step Delta Time"=1150198, "Measurement -> Sense"=1150013, "Measurement -> Aperture Time"=1150058, "Measurement -> Measure Record Length"=1150063, "Measurement -> Advanced -> DC Noise Rejection"=1150066, "Measurement -> Autorange"=1150244, "Measurement -> Advanced -> Autorange Behavior"=1150245, "Measurement -> Advanced -> Autorange Aperture Time Mode"=1150246, "Measurement -> Advanced -> Autorange Minimum Aperture Time"=1150247, "Measurement -> Advanced -> Autorange Minimum Aperture Time Units"=1150248, "Measurement -> Advanced -> Autorange Minimum Current Range"=1150255, "Measurement -> Advanced -> Autorange Minimum Voltage Range"=1150256, "Measurement -> Advanced -> Autorange Threshold Mode"=1150257, "Measurement -> Advanced -> Autorange Maximum Delay After Range Change"=1150322, "LCR -> Instrument Mode"=1150208, "LCR -> LCR Stimulus Function"=1150209, "LCR -> LCR Frequency"=1150210, "LCR -> LCR Voltage Amplitude"=1150211, "LCR -> LCR Current Amplitude"=1150212, "LCR -> LCR DC Bias Source"=1150213, "LCR -> LCR DC Bias Voltage Level"=1150214, "LCR -> LCR DC Bias Current Level"=1150215, "LCR -> LCR Impedance Autorange"=1150216, "LCR -> LCR Impedance Range"=1150217, "LCR -> LCR Measurement Time"=1150218, "LCR -> LCR Custom Measurement Time"=1150258, "LCR -> LCR Source Delay Mode"=1150315, "LCR -> Compensation -> Open -> Enabled"=1150220, "LCR -> Compensation -> Open -> Conductance"=1150261, "LCR -> Compensation -> Open -> Susceptance"=1150262, "LCR -> Compensation -> Short -> Enabled"=1150221, "LCR -> Compensation -> Short -> Resistance"=1150263, "LCR -> Compensation -> Short -> Reactance"=1150264, "LCR -> Compensation -> Load -> Enabled"=1150222, "LCR -> Compensation -> Load -> Measured Resistance"=1150268, "LCR -> Compensation -> Load -> Measured Reactance"=1150269, "LCR -> Compensation -> Load -> Actual Resistance"=1150270, "LCR -> Compensation -> Load -> Actual Reactance"=1150271] ("advanced sequence properties")
            w210 = "SourceVoltages" ("sequence name")
            w197 = T9 1006 items=["DC Voltage"=1006, "DC Current"=1007, "Pulse Voltage"=1049, "Pulse Current"=1050] ("output function")
            w196 = T6 1021 items=["Single Point"=1020, "Sequence"=1021] ("source mode")
            # "1. Configuring the source to sequence as we are plotting for multiple voltages.\n2. Advanced sequencing is used as the current limit values are also modified along with voltage values.\n3. Acquires a measurement automatically after every source operation and stores it in a buffer on the device."
            n65 = Unbundle By Name(w221) -> ("Source delay"=w219:dbl, "Source current limit"=w218:dbl, "Source maximum power"=w217:dbl, "Aperture time"=w216:dbl)
            n66 = Unbundle By Name(w223) -> ("Load sweep points"=w214:i32, "Source channel name"=w213:string, "Source out"=w215:refnum<k15>, "Voltage values"=w212:dbl[])
            n67 = call <instrlib>:"niDCPower Configure Source Mode With Channels.vi"("error in (no error)"=w220, "source mode"=w196, "channel name"=w213, "instrument handle"=w215) -> ("error out"=w194:errorcluster, "instrument handle out"=w195:refnum<k15>)  [unwired: 6 in]
            n68 = call <instrlib>:"niDCPower Configure Output Function.vi"("error in (no error)"=w194, "output function"=w197, "channel name"=w213, "instrument handle"=w195) -> ("error out"=w205:errorcluster, "instrument handle out"=w204:refnum<k15>)  [unwired: 6 out]
            n69 = property class="niDCPower"(reference=w204, error in=w205, "Active Channel"=w213, "Source:DC Voltage:Voltage Level Autorange"=w201, "Source:DC Voltage:Current Limit Autorange"=w201) -> (reference out=w202:refnum<k15>, error out=w203:errorcluster)
            n70 = property class="niDCPower"(reference=w202, error in=w203, "Active Channel"=w213, "Source Delay"=w219) -> (reference out=w208:refnum<k15>, error out=w209:errorcluster)
            n71 = call <instrlib>:"niDCPower Create Advanced Sequence With Channels.vi"("instrument handle"=w208, "channel name"=w213, "sequence name"=w210, "advanced sequence properties"=w200, "error in (no error)"=w209) -> ("instrument handle out"=w198:refnum<k15>, "error out"=w199:errorcluster)  [unwired: 9 in]
            n72 = for {
              tunnel: w217 -> [w228]
              tunnel: w218 -> [w227]
              tunnel: w212 -> [w226] mode=indexing
              shift-right: [w230] -> w206
              shift-left: w198 -> [w232]
              shift-right: [w229] -> w207
              shift-left: w199 -> [w231]
              tunnel: w214 -> [w225]
              tunnel: w213 -> [w224]
              n73 = for {
                N: w225 -> [_]
                shift-right: [w240] -> w229
                shift-left: w231 -> [w243]
                shift-right: [w239] -> w230
                shift-left: w232 -> [w238]
                tunnel: w228 -> [w235]
                tunnel: w226 -> [w233]
                tunnel: w227 -> [w236]
                tunnel: w224 -> [w237]
                n74 = call-poly <instrlib>:"niDCPower Create Advanced Sequence Step With Channels (Poly).vi"("error in (no error)"=w243, "channel name"=w237, "instrument handle"=w238) -> ("error out"=w241:errorcluster, "instrument handle out"=w242:refnum<k15>)  [unwired: 7 in]
                n75 = call "Calculate Current Limit.vi"("Voltage value"=w233, "Maximum power"=w235, "Current limit in"=w236) -> ("Current limit out"=w234:dbl)  [unwired: 8 in]
                n76 = property class="niDCPower"(reference=w242, error in=w241, "Voltage Level"=w233, "Current Limit"=w234) -> (reference out=w239:refnum<k15>, error out=w240:errorcluster)
              }
            }
            n77 = property class="niDCPower"(reference=w206, error in=w207, "Measure When"=w193, "Aperture Time"=w216) -> (reference out=w191:refnum<k15>, error out=w192:errorcluster)
            n78 = call <instrlib>:"niDCPower Commit With Channels.vi"("error in (no error)"=w192, "channel name"=w213, "instrument handle"=w191) -> ("error out"=w211:errorcluster, "instrument handle out"=w190:refnum<k15>)  [unwired: 7 in]
            n79 = Bundle By Name(cluster=w223, "Source sequence name"=w210, "Source out"=w190) -> (w222:T3)
          }
          frame "ConfigureLoadToSequence" {
            w251 = T9 1007 items=["DC Voltage"=1006, "DC Current"=1007, "Pulse Voltage"=1049, "Pulse Current"=1050] ("output function")
            w250 = 1027 items=["Automatically after Source Complete"=1025, "On Demand"=1026, "On Measure Trigger"=1027] ("Measurement:Advanced:Measure When")
            w249 = T6 1021 items=["Single Point"=1020, "Sequence"=1021] ("source mode")
            # "1. Configuring the load to sequence as we are sweeping load currents\n2. Set the current sequence\n3. Acquires a measurement when it receives a Measure trigger. \nSo, when a 'SourceCompleteEvent' occurs in the source device, the load device will start acquiring the measurement."
            n80 = Unbundle By Name(w267) -> ("Aperture time"=w266:dbl)
            n81 = Unbundle By Name(w263) -> ("Load channel name"=w272:string, "Load out"=w271:refnum<k15>)
            n82 = Unbundle By Name(w263) -> ("Current values"=w270:dbl[], "Source terminal name"=w269:string, "Measure terminal name"=w268:string)
            n83 = call <instrlib>:"niDCPower Configure Source Mode With Channels.vi"("error in (no error)"=w273, "source mode"=w249, "channel name"=w272, "instrument handle"=w271) -> ("error out"=w247:errorcluster, "instrument handle out"=w248:refnum<k15>)  [unwired: 6 in]
            n84 = call <instrlib>:"niDCPower Configure Output Function.vi"("error in (no error)"=w247, "output function"=w251, "channel name"=w272, "instrument handle"=w248) -> ("error out"=w260:errorcluster, "instrument handle out"=w259:refnum<k15>)  [unwired: 6 out]
            n85 = call <instrlib>:"niDCPower Set Sequence.vi"("error in (no error)"=w260, "values"=w270, "channel name"=w272, "instrument handle"=w259) -> ("error out"=w255:errorcluster, "instrument handle out"=w254:refnum<k15>)  [unwired: 1 in, 5 out]
            n86 = property class="niDCPower"(reference=w254, error in=w255, "Active Channel"=w272, "Source Delay"=0.0 ("Source:Advanced:Source Delay")) -> (reference out=w252:refnum<k15>, error out=w253:errorcluster)
            n87 = call-poly <instrlib>:"niDCPower Configure Trigger With Channels (Poly).vi"("error in (no error)"=w253, "input terminal"=w269, "channel name"=w272, "instrument handle"=w252) -> ("error out"=w244:errorcluster, "instrument handle out"=w261:refnum<k15>)  [unwired: 6 in]
            n88 = property class="niDCPower"(reference=w261, error in=w244, "Measure When"=w250, "Aperture Time"=w266) -> (reference out=w246:refnum<k15>, error out=w245:errorcluster)
            n89 = call-poly <instrlib>:"niDCPower Configure Trigger With Channels (Poly).vi"("error in (no error)"=w245, "input terminal"=w268, "channel name"=w272, "instrument handle"=w246) -> ("error out"=w256:errorcluster, "instrument handle out"=w257:refnum<k15>)  [unwired: 6 in]
            n90 = call <instrlib>:"niDCPower Commit With Channels.vi"("error in (no error)"=w256, "channel name"=w272, "instrument handle"=w257) -> ("error out"=w265:errorcluster, "instrument handle out"=w264:refnum<k15>)  [unwired: 7 in]
            n91 = Bundle By Name(cluster=w263, "Load out"=w264) -> (w262:T3)
          }
          frame "StartSourceAndLoad" {
            # "Start the load and source device and waits for all the sequences to be completed within 10 sec (default)."
            n92 = Unbundle By Name(w278) -> ("Source out"=w283:refnum<k15>, "Source channel name"=w280:string, "Load out"=w282:refnum<k15>, "Load channel name"=w281:string)
            n93 = flat-sequence {
              tunnel: [w295] -> w287
              tunnel: [w294] -> w286
              tunnel: [w293] -> w285
              tunnel: w279 -> [w292]
              tunnel: w282 -> [w291]
              tunnel: w283 -> [w290]
              tunnel: w280 -> [w289]
              tunnel: [w288] -> w284
              tunnel: w281 -> [w288]
              tunnel: w287 -> [w303]
              tunnel: w286 -> [w301]
              tunnel: w285 -> [w298]
              tunnel: [w303] -> w277
              tunnel: [w299] -> w274
              tunnel: [w300] -> w276
              tunnel: w284 -> [w297]
              frame #0 {
                n94 = call <instrlib>:"niDCPower Initiate With Channels.vi"("error in (no error)"=w292, "channel name"=w288, "instrument handle"=w291) -> ("error out"=w296:errorcluster, "instrument handle out"=w293:refnum<k15>)  [unwired: 7 in]
                n95 = call <instrlib>:"niDCPower Initiate With Channels.vi"("error in (no error)"=w296, "channel name"=w289, "instrument handle"=w290) -> ("error out"=w294:errorcluster, "instrument handle out"=w295:refnum<k15>)  [unwired: 7 in]
              }
              frame #1 {
                w302 = T5 1033 items=["Source Complete Event"=1030, "Measure Complete Event"=1031, "Sequence Iteration Complete Event"=1032, "Sequence Engine Done Event"=1033] ("event")
                n96 = call <instrlib>:"niDCPower Wait For Event With Channels.vi"("error in (no error)"=w301, "event"=w302, "channel name"=w297, "instrument handle"=w298) -> ("error out"=w299:errorcluster, "instrument handle out"=w300:refnum<k15>)  [unwired: 6 in]
              }
            }
            n97 = Bundle By Name(cluster=w278, "Source out"=w277, "Load out"=w276) -> (w275:T3)
          }
          frame "PerformMeasurement" {
            # "1.Fetches the voltages and currents of both the PPS and E-Load\n2.Calculates the efficiency (%), load voltage deviation (%)"
            n98 = Unbundle By Name(w311) -> ("Nominal output voltage"=w307:dbl)
            n99 = call "Perform Measurements.vi"("error in"=w313, "Measurement Context"=w305, "Nominal output voltage"=w307, "Reference values"=w306) -> ("error out"=w312:errorcluster, "Measurement Results"=w308:T1, "Load out"=w309:refnum<k15>, "Source out"=w310:refnum<k15>)  [unwired: 3 in]
            n100 = Bundle By Name(cluster=w306, "Source out"=w310, "Load out"=w309, "Measurement Results"=w308) -> (w304:T3)
          }
          frame "Exit", Default {
            # "1. Aborts the channels\n2. Deletes the created advanced sequence\n3. Close all the opened sessions"
            n101 = Release Queue(queue=w315, error in (no error)=w320) -> (error out=w319:errorcluster)  [unwired: 1 in, 2 out]
            n102 = case shown="No Error" w319 {
              selector: w319 -> [w322 w353]
              tunnel: [w321 w352] -> w317
              tunnel: w318 -> [w323 w351]
              tunnel: [w336 w351] -> w316
              frame No Error {
                # "Updates the status indicator on the operation performed if there is no error"
                n103 = Unbundle By Name(w323) -> ("Source out"=w334:refnum<k15>, "Source channel name"=w328:string, "Source sequence name"=w324:string, "Load out"=w333:refnum<k15>, "Load channel name"=w332:string)
                n104 = call <instrlib>:"niDCPower Abort With Channels.vi"("error in (no error)"=w322, "channel name"=w332, "instrument handle"=w333) -> ("error out"=w335:errorcluster, "instrument handle out"=w325:refnum<k15>)  [unwired: 7 in]
                n105 = call <instrlib>:"niDCPower Close.vi"("error in (no error)"=w335, "instrument handle"=w325) -> ("error out"=w327:errorcluster)  [unwired: 9 in]
                n106 = call <instrlib>:"niDCPower Abort With Channels.vi"("error in (no error)"=w327, "channel name"=w328, "instrument handle"=w334) -> ("error out"=w330:errorcluster, "instrument handle out"=w329:refnum<k15>)  [unwired: 7 in]
                n107 = call <instrlib>:"niDCPower Delete Advanced Sequence With Channels.vi"("error in (no error)"=w330, "sequence name"=w324, "channel name"=w328, "instrument handle"=w329) -> ("error out"=w331:errorcluster, "instrument handle out"=w326:refnum<k15>)  [unwired: 6 in]
                n108 = call <instrlib>:"niDCPower Close.vi"("error in (no error)"=w331, "instrument handle"=w326) -> ("error out"=w321:errorcluster)  [unwired: 9 in]
                n109 = Bundle By Name(cluster=w323, "Measurement Results.Status"="The measurement is performed successfully" ("message")) -> (w336:T3)
              }
              frame Error {
                # "Resets the device with default values whenever there is an error"
                n110 = Unbundle By Name(w351) -> ("Source out"=w342:refnum<k15>, "Source channel name"=w340:string, "Load out"=w339:refnum<k15>, "Load channel name"=w338:string)
                n111 = call <instrlib>:"niDCPower Abort With Channels.vi"("error in (no error)"=w353, "channel name"=w338, "instrument handle"=w339) -> ("error out"=w346:errorcluster, "instrument handle out"=w343:refnum<k15>)  [unwired: 7 in]
                n112 = call <instrlib>:"niDCPower Reset With Channels.vi"("error in (no error)"=w346, "channel name"=w338, "instrument handle"=w343) -> ("error out"=w347:errorcluster, "instrument handle out"=w348:refnum<k15>)  [unwired: 7 in]
                n113 = call <instrlib>:"niDCPower Close.vi"("error in (no error)"=w347, "instrument handle"=w348) -> ("error out"=w341:errorcluster)  [unwired: 9 out]
                n114 = call <instrlib>:"niDCPower Abort With Channels.vi"("error in (no error)"=w341, "channel name"=w340, "instrument handle"=w342) -> ("error out"=w344:errorcluster, "instrument handle out"=w345:refnum<k15>)  [unwired: 7 in]
                n115 = call <instrlib>:"niDCPower Reset With Channels.vi"("error in (no error)"=w344, "channel name"=w340, "instrument handle"=w345) -> ("error out"=w350:errorcluster, "instrument handle out"=w349:refnum<k15>)  [unwired: 7 in]
                n116 = call <instrlib>:"niDCPower Close.vi"("error in (no error)"=w350, "instrument handle"=w349) -> ("error out"=w352:errorcluster)  [unwired: 9 out]
              }
            }
          }
        }
      }
    }
    frame "Power off the DUT" {
      # "Stops generation on the output channel and resets the channels to default values"
      n117 = Unbundle By Name(w372) -> ("Source resource name"=w374:string, "Load resource name"=w377:string)
      n118 = call <instrlib>:"niDCPower Initialize With Independent Channels.vi"("error in (no error)"=w384, "resource name"=w377) -> ("error out"=w378:errorcluster, "instrument handle out"=w376:refnum<k15>)  [unwired: 8 in]
      n119 = call-poly <instrlib>:"niDCPower Get Channel Name (Poly).vi"("error in (no error)"=w378, "index"="0", "instrument handle"=w376) -> ("error out"=w389:errorcluster, "name"=w386:string, "instrument handle out"=w387:refnum<k15>)  [unwired: 6 in]
      n120 = call <instrlib>:"niDCPower Configure Output Enabled.vi"("error in (no error)"=w389, "output enabled"=FALSE, "channel name"=w386, "instrument handle"=w387) -> ("error out"=w396:errorcluster, "instrument handle out"=w395:refnum<k15>)  [unwired: 6 in]
      n121 = call <instrlib>:"niDCPower Reset With Channels.vi"("error in (no error)"=w396, "channel name"=w386, "instrument handle"=w395) -> ("error out"=w390:errorcluster, "instrument handle out"=w391:refnum<k15>)  [unwired: 7 in]
      n122 = call <instrlib>:"niDCPower Close.vi"("error in (no error)"=w390, "instrument handle"=w391) -> ("error out"=w381:errorcluster)  [unwired: 9 out]
      n123 = call <instrlib>:"niDCPower Initialize With Independent Channels.vi"("error in (no error)"=w381, "resource name"=w374) -> ("error out"=w375:errorcluster, "instrument handle out"=w373:refnum<k15>)  [unwired: 8 in]
      n124 = call-poly <instrlib>:"niDCPower Get Channel Name (Poly).vi"("error in (no error)"=w375, "index"="0", "instrument handle"=w373) -> ("error out"=w380:errorcluster, "name"=w379:string, "instrument handle out"=w382:refnum<k15>)  [unwired: 6 in]
      n125 = call <instrlib>:"niDCPower Reset With Channels.vi"("error in (no error)"=w380, "channel name"=w379, "instrument handle"=w382) -> ("error out"=w393:errorcluster, "instrument handle out"=w392:refnum<k15>)  [unwired: 7 in]
      n126 = call <instrlib>:"niDCPower Close.vi"("error in (no error)"=w393, "instrument handle"=w392) -> ("error out"=w385:errorcluster)  [unwired: 9 out]
      n127 = Bundle By Name(cluster=w370, "Measurement Results.Status"="The DUT is powered OFF") -> (w368:T3)
    }
  }
  "error out" <- w1
  "measure call context out" <- w3
  n128 = Unbundle By Name(w2) -> ("Measurement Results"=→"measurement results":T1)
